vi "Vision-Goal.vi"() -> (12 "Goal Detected":bool, 14 "Goal Angle (radians 0=right)":dbl, 15 "Goal Distance (from front of shooter)":dbl)   [LabVIEW 2015]
uses:
  Team900-VIs/labview-zmq/socket_type.ctl
  Team900-VIs/labview-zmq/socket_options.ctl
  Team900-VIs/labview-zmq/zmq_socket.lvclass
  Team900-VIs/labview-zmq/zmq_context.lvclass
  Team900-VIs/labview-zmq/zeromq.lvlib
panel:
  in  "Reset":bool
  out "data 2":string
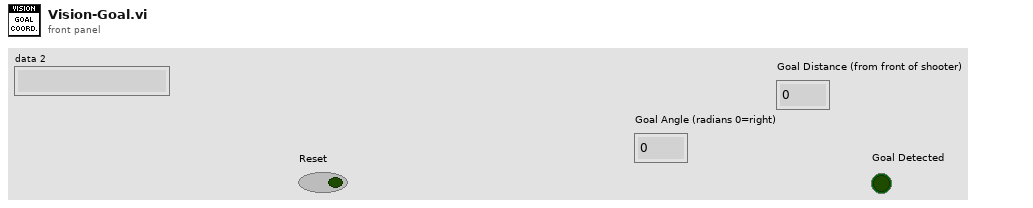
[diagram p1: front panel]
types:
  T1 = typedef "zeromq.lvlib/socket_options.ctl" = enum8{"NONE", "ZMQ_HWM", "<2>", "ZMQ_SWAP", "ZMQ_AFFINITY", "ZMQ_IDENTITY", "ZMQ_SUBSCRIBE", "ZMQ_UNSUBSCRIBE", "ZMQ_RATE", "ZMQ_RECOVERY_IVL", "ZMQ_MCAST_LOOP", "ZMQ_SNDBUF", "ZMQ_RCVBUF", "ZMQ_RCVMORE", "ZMQ_FD", "ZMQ_EVENTS", "ZMQ_TYPE", "ZMQ_LINGER", "ZMQ_RECONNECT_IVL", "ZMQ_BACKLOG", "ZMQ_RECOVERY_IVL_MSEC", "ZMQ_RECONNECT_IVL_MAX", "ZMQ_MAXMSGSIZE", "ZMQ_SNDHWM", "ZMQ_RCVHWM", "ZMQ_MULTICAST_HOPS", "<26>", "ZMQ_RCVTIMEO", "ZMQ_SNDTIMEO", "<29>", "<30>", "ZMQ_IPV4ONLY", "ZMQ_LAST_ENDPOINT", "ZMQ_ROUTER_MANDATORY", "ZMQ_TCP_KEEPALIVE", "ZMQ_TCP_KEEPALIVE_CNT", "ZMQ_TCP_KEEPALIVE_IDLE", "ZMQ_TCP_KEEPALIVE_INTVL", "ZMQ_TCP_ACCEPT_FILTER", "ZMQ_DELAY_ATTACH_ON_CONNECT", "ZMQ_XPUB_VERBOSE"}
  T2 = typedef "zeromq.lvlib/socket_type.ctl" = enum8{"ZMQ_PAIR", "ZMQ_PUB", "ZMQ_SUB", "ZMQ_REQ", "ZMQ_REP", "ZMQ_DEALER", "ZMQ_ROUTER", "ZMQ_PULL", "ZMQ_PUSH", "ZMQ_XPUB", "ZMQ_XSUB"}
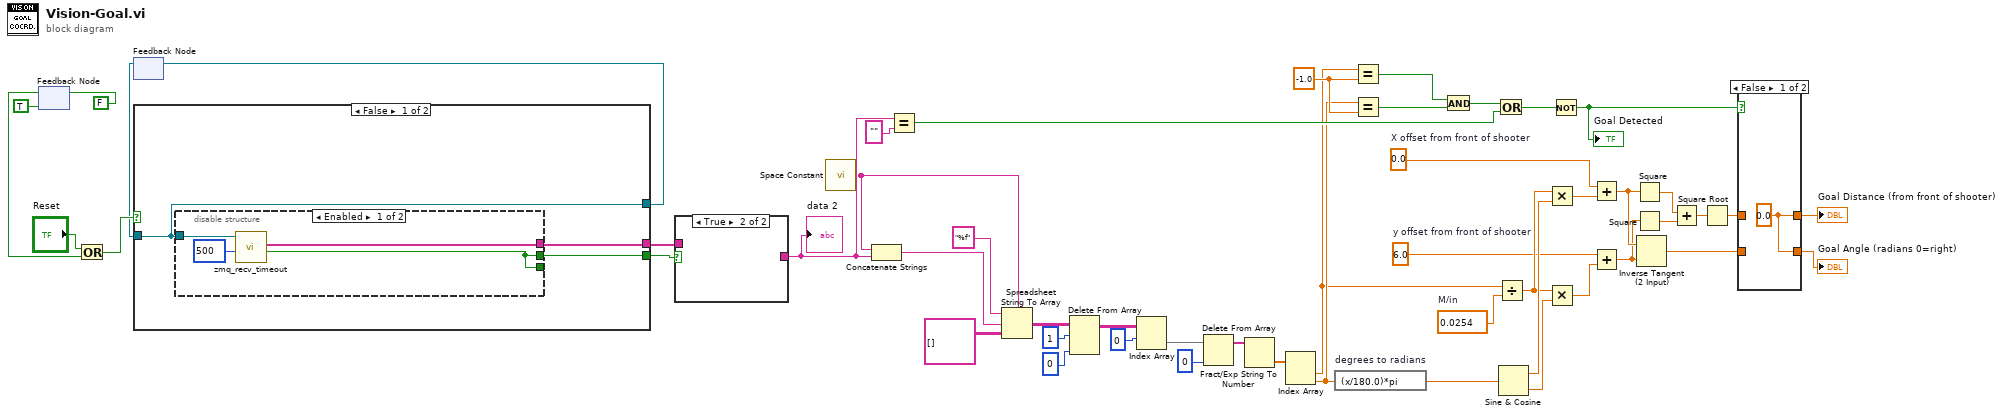
[diagram p0: block diagram]
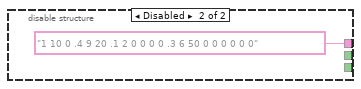
[diagram p2: hidden frame]
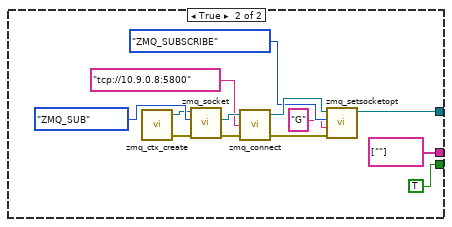
[diagram p3: hidden frame]
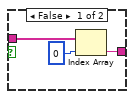
[diagram p4: hidden frame]
diagram:
  w38 = 6.0  # y offset from front of shooter
  w39 = 0.0  # X offset from front of shooter
  w51 = 0.0254  # M/in
  w26 = -1.0 ("y")
  n1 = feedback #1(TRUE) -> (w18:bool)
  n2 = feedback-in #1(FALSE) -> ()
  n3 = Or(x="Reset", y=w18) -> (x .or. y?=w33:bool)
  n4 = feedback #2() -> (w6:refnum<class "zmq_socket.lvclass">)  [unwired: 1 in]
  n5 = case shown="False" w33 {
    tunnel: [w54 string[] [""] ("parts")] -> w9
    tunnel: [w53 TRUE ("timeout?")] -> w8
    tunnel: w6 -> [w52 _]
    tunnel: [w52 w60] -> w7
    frame False {
      n6 = disable-structure shown="Enabled" {
        disable-tunnel: [w58 "1 10 0 .4 9 20 .1 2 0 0 0 0 .3 6 50 0 0 0 0 0 0"] -> w54
        disable-tunnel: [w56 _] -> w53
        disable-tunnel: [w56 _] -> _
        disable-tunnel: w52 -> [w55 _]
        frame Enabled {
          n7 = call "zmq_recv_timeout.vi"("timeout (ms)"=u32 500, "socket in"=w55) -> ("timeout?"=w56:bool, "parts"=w58:string[])  [unwired: 2 in, 2 out]
        }
        frame Disabled {
        }
      }
    }
    frame True {
      n8 = call "zmq_ctx_create.vi"() -> ("error out"=w68:errorcluster, "context out"=w71:refnum<class "zmq_context.lvclass">)  [unwired: 4 in]
      n9 = call "zmq_socket.vi"("error in"=w68, "socket type"=socket_type."ZMQ_SUB", "context in"=w71) -> ("error out"=w65:errorcluster, "socket out"=w70:refnum<class "zmq_socket.lvclass">)  [unwired: 2 in, 1 out]
      n10 = call "zmq_connect.vi"("error in"=w65, "endpoint"="tcp://10.9.0.8:5800" ("Endpoint"), "socket in"=w70) -> ("error out"=w66:errorcluster, "socket out"=w67:refnum<class "zmq_socket.lvclass">)  [unwired: 1 in]
      n11 = call "zmq_setsocketopt.vi"("error in"=w66, "value"="G", "option"=socket_options."ZMQ_SUBSCRIBE", "socket in"=w67) -> ("socket out"=w60:refnum<class "zmq_socket.lvclass">)  [unwired: 2 in, 1 out]
    }
  }
  n12 = feedback-in #2(w7) -> ()
  n13 = case shown="True" w8 {
    tunnel: w9 -> [w75 _]
    tunnel: [w73 _] -> w37
    frame False {
      n14 = Index Array(array=w75, index=0) -> (element=w73:string)
    }
    frame True {
    }
  }
  "data 2" <- w37
  n15 = call <vilib>:"Space Constant.vi"() -> ("String"=w10:string)
  n16 = Concatenate Strings(w10, w37) -> (w11:string)
  n17 = Equal?(x=w37, y="") -> (x = y?=w35:bool)
  n18 = Spreadsheet String To Array(delimiter (Tab)=w10, format string="%f", spreadsheet string=w11, array type (2D Dbl)=string[][] [] ("Array")) -> (array=w12:string[][])
  n19 = Delete From Array(array=w12, length=1, index (col)=0 ("disabled index (col)")) -> (array with subset deleted=w5:string[][])  [unwired: 1 in, 1 out]
  n20 = Index Array(array=w5, index (row)=0) -> (element=w2:string[])  [unwired: 1 in]
  n21 = Delete From Array(array=w2, index=0) -> (array with subset deleted=w1:string[])  [unwired: 1 in, 1 out]
  n22 = Fract/Exp String To Number(string=w1) -> (number=w32:dbl[])  [unwired: 4 out]
  n23 = Index Array(array=w32) -> (element #1=w21:dbl, element #2=w22:dbl)  [unwired: 2 in]
  n24 = expression code="(x/180.0)*pi" "degrees to radians"(w22) -> (w50:dbl)
  n25 = Equal?(x=w21, y=w26) -> (x = y?=w24:bool)
  n26 = Equal?(x=w22, y=w26) -> (x = y?=w25:bool)
  n27 = And(x=w24, y=w25) -> (x .and. y?=w23:bool)
  n28 = Or(x=w23, y=w35) -> (x .or. y?=w34:bool)
  n29 = Divide(x=w21, y=w51) -> (x/y=w46:dbl)
  n30 = Sine & Cosine(0:w50) -> (1:w49:dbl, 2:w47:dbl)
  n31 = Multiply(x=w46, y=w49) -> (x*y=w48:dbl)
  n32 = Multiply(x=w46, y=w47) -> (x*y=w45:dbl)
  n33 = Not(x=w34) -> (.not. x?=w27:bool)
  "Goal Detected" <- w27
  n34 = Add(x=w39, y=w48) -> (x+y=w41:dbl)
  n35 = Add(x=w38, y=w45) -> (x+y=w40:dbl)
  n36 = Square(x=w41) -> (x^2=w44:dbl)
  n37 = Square(x=w40) -> (x^2=w43:dbl)
  n38 = Inverse Tangent (2 Input)(1:w40, 2:w41) -> (0:w30:dbl)
  n39 = Add(x=w44, y=w43) -> (x+y=w42:dbl)
  n40 = Square Root(x=w42) -> (sqrt(x)=w28:dbl)
  n41 = case shown="False" w27 {
    tunnel: [w76 w78] -> w31
    tunnel: w30 -> [_ w78]
    tunnel: [w76 w77] -> w29
    tunnel: w28 -> [_ w77]
    frame False {
      w76 = 0.0
    }
    frame True {
    }
  }
  "Goal Distance (from front of shooter)" <- w29
  "Goal Angle (radians 0=right)" <- w31
